vi "sample_calibration_sort_centroids.vi"(8 "Error In":errorcluster, 11 "centroids":sgl[][](array[numeric])) -> (0 "Error Out":errorcluster, 2 "Right Centroids":dbl[][](array[numeric]), 3 "Left Centroids":dbl[][](array[numeric]))   [LabVIEW 2019]
uses:
  6e857618-e883-4d80-845c-368e6bbf1c5b.vi
  6528a5fc-19e9-4b5c-8562-3b78e73d9c40.vi
  4c631271-7f91-4e3a-8e6b-63f1b0d1ace1.vi
  <vilib>/Array/Sort 2D Array - Pop Stack.vi
  <vilib>/Array/Sort 2D Array - Push Stack.vi
  6e857618-e883-4d80-845c-368e6bbf1c5b.vi/e4906d37-f3f9-4ccf-a178-05a7e0dbd239.vi
  6e857618-e883-4d80-845c-368e6bbf1c5b.vi/82dacc78-74b3-4b21-9107-91da41ac0e82.vi
  6528a5fc-19e9-4b5c-8562-3b78e73d9c40.vi/578df5b2-b93f-4f59-8118-793ee723797a.vi
  6528a5fc-19e9-4b5c-8562-3b78e73d9c40.vi/daa2a90b-7d8b-4d2c-a8a0-21f5e19d6cfa.vi
  4c631271-7f91-4e3a-8e6b-63f1b0d1ace1.vi/b1a43179-d613-44f4-a2a0-7278b41c91e9.vi
  4c631271-7f91-4e3a-8e6b-63f1b0d1ace1.vi/7bd7700a-ee4f-4db5-91e8-fb6fd50f3548.vi
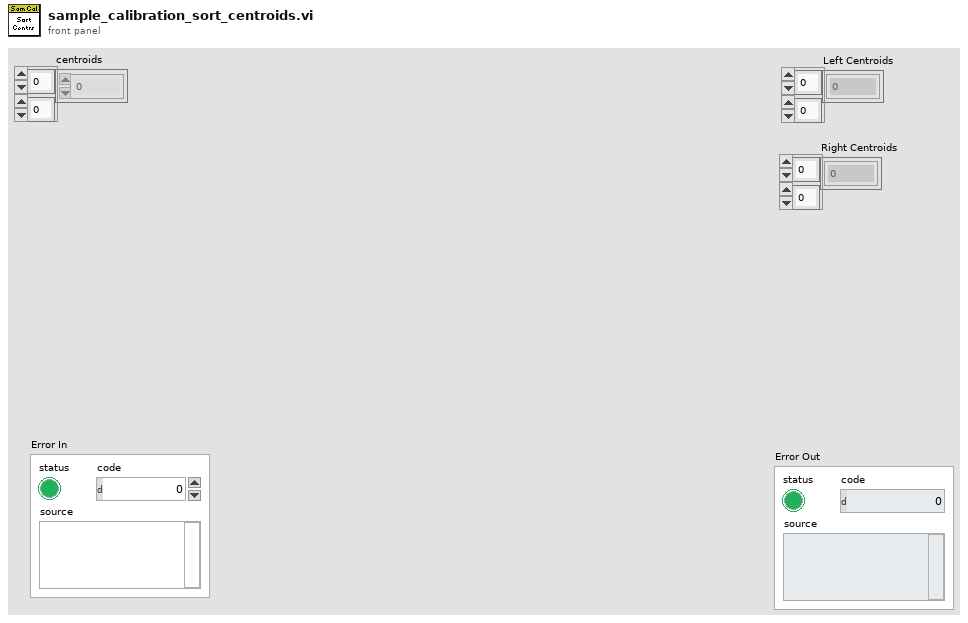
[diagram p1: front panel]
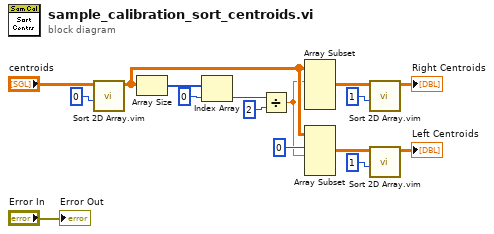
[diagram p0: block diagram]
diagram:
  n1 = call "Sort 2D Array.vim"("index"=0, "2D array"="centroids") -> ("sorted 2D array"=w10:sgl[][])  [unwired: 8 in, 1 out]
  n2 = Array Size(array=w10) -> (size(s)=w15:i32[])
  n3 = Index Array(array=w15, index=0) -> (element=w13:i32)
  n4 = Divide(x=w13, y=2) -> (x/y=w9:dbl)
  n5 = Array Subset(array=w10, index (row)=w9) -> (w6:sgl[][])  [unwired: 3 in]
  n6 = Array Subset(array=w10, index (row)=0 ("index"), length (row)=w9) -> (w8:sgl[][])  [unwired: 2 in]
  n7 = call "Sort 2D Array.vim"("index"=1, "2D array"=w6) -> ("sorted 2D array"=→"Right Centroids":sgl[][])  [unwired: 8 in, 1 out]
  n8 = call "Sort 2D Array.vim"("index"=1, "2D array"=w8) -> ("sorted 2D array"=→"Left Centroids":sgl[][])  [unwired: 8 in, 1 out]
  "Error Out" <- "Error In"
